vi "Log Data.vi"(8 "error in (no error)":errorcluster, 11 "OD600 in":refnum<class "OD600.lvclass">) -> (0 "error out":errorcluster, 3 "OD600 out":refnum<class "OD600.lvclass">)   [LabVIEW 2013, in "OD600.lvlib" / "OD600.lvclass"]
uses:
  OD600.lvclass
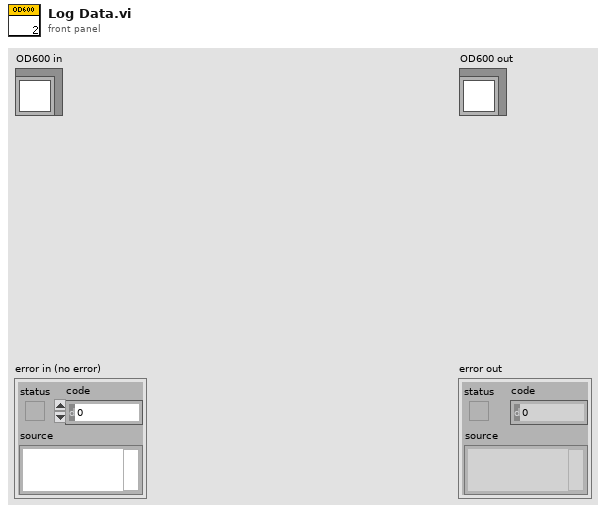
[diagram p1: front panel]
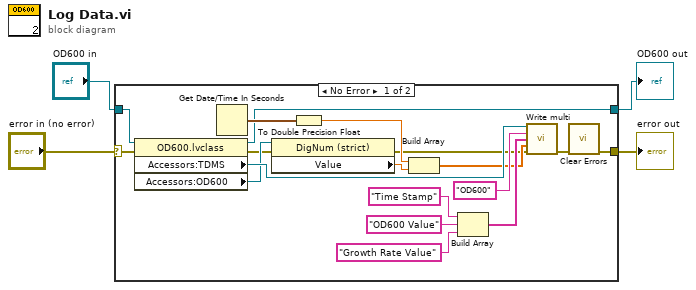
[diagram p0: block diagram]
diagram:
  n1 = case shown="No Error" "error in (no error)" {
    selector: "error in (no error)" -> [w13 w24]
    tunnel: [w6 w24] -> w1
    tunnel: [w20 w23] -> w2
    tunnel: "OD600 in" -> [w21 w23]
    frame No Error {
      n2 = property class="OD600.lvclass"(reference=w21, error in=w13) -> (reference out=w20:refnum<class "OD600.lvclass">, error out=w9:errorcluster, "Accessors:TDMS"=w19:refnum<k34>, "Accessors:OD600"=w10:refnum<vi>)
      n3 = Get Date/Time In Seconds() -> (seconds since 1Jan1904=w22:timestamp)
      n4 = property class="DigNum (strict)"(reference=w10, error in=w9) -> (error out=w8:errorcluster, "Value"=w12:dbl)  [unwired: 1 out]
      n5 = To Double Precision Float(number=w22) -> (double precision float=w14:dbl)
      n6 = Build Array(w14, w12) -> (w11:dbl[])
      n7 = Build Array("Time Stamp" ("Channel"), "OD600 Value" ("string"), "Growth Rate Value" ("string")) -> (w15:string[])
      n8 = call "Write multi.vi"("tdms file in"=w19, "group"="OD600", "Channel"=w15, "Data"=w11, "error in (no error)"=w8) -> ("error out"=w7:errorcluster)  [unwired: 7 in, 3 out]
      n9 = call <vilib>:"Clear Errors.vi"("error in (no error)"=w7) -> ("error out"=w6:errorcluster)  [unwired: 6 in]
    }
    frame Error {
    }
  }
  "error out" <- w1
  "OD600 out" <- w2
